vi "Analysis Configuration Dialog.vi"(11 "Data in":T1={"UI References"={"Stop Ref"=refnum, "Save Ref"=refnum, "Open Ref"=refnum, "Export Ref"=refnum, "Acquire Ref"=refnum, "Configure Ref"=refnum, "Graph Ref"=refnum, "Clear Ref"=refnum, "Analyze Ref"=refnum, "Status Ref"=refnum, "Snapshot Ref"=refnum}, "Graph Data"={"Data"=[{"t0"=timestamp(0 s since 1904-01-01), "dt"=0.001, "Y"=[0.0, 0.18799846683964833, 0.3692926533087303, 0.5374173627698757, 0.6863770400018341, 0.8108595808323735, 0.9064257689795854, 0.9696675845268409, 0.9983297385364166, 0.9913900997125904, 0.9490961449902946, 0.8729561341718822, 0.7656853233364365, 0.6311091351244097, 0.47402673897660996, 0.300039906241276, 0.11535324340830803, -0.07344707257547595, -0.25962816631122254, -0.4365505674187408, -0.5979049830575192, -0.7379372958687495, -0.8516537636065122, -0.9349991027608904, -0.9850011054694262, -0.9998766324816605, -0.9790952023238538, -0.9233979089880013, -0.8347709935146953, -0.716375011943035, -0.5724321255945906, -0.40807553307279343, -0.22916641343692226, -0.04208490860543837, 0.1464974011602751, 0.3298554148588533, 0.5014503369740866, 0.655162859793709, 0.7855113862240124, 0.887847510978669, 0.9585217890173761, 0.9950138797069145, 0.9960224255872819, 0.9615114605441677, 0.8927116924093821, 0.7920766142499667, 0.663195009476959, 0.5106629709603275, 0.33991999812206386, 0.15705501700744282, -0.03141075907812895, -0.21875638488241306, -0.39830086123182346, -0.5636413885255546, -0.7088816992555318, -0.8288423269047623, -0.9192453127499152, -0.9768667636729723, -0.9996518205634258, -0.9867879373818272, -0.9387338576538738, -0.8572032550539391, -0.7451036214770367, -0.6064325819334717, -0.44613533381770504, -0.26992829446049543, -0.0840952459318628, 0.1047367531522541, 0.28983369753066196, 0.46459477906003466, 0.6227877804881133, 0.758771324775691, 0.8676960542550545, 0.9456775653031642, 0.9899349314445249, 0.9988898749619699, 0.972223050421184, 0.9108854329621217, 0.8170644052354027, 0.6941057523695359, 0.5463943467342681, 0.37919777744325917, 0.1984785009801561, 0.010681211911579646, -0.17749698366414263, -0.3593453960058918, -0.5283790640298028, -0.6785700178191627, -0.8045622442093244, -0.9018626894832488, -0.9670014877624354, -0.9976557011314492, -0.9927321587553373, -0.9524064408346227, -0.8781166171771593, -0.7725119636778635, -0.6393584855462336, -0.483404616451529, -0.3102118829362894, -0.12595657283493283], "attributes"=variant("NI_ChannelName"=variant(string "Sine"), "NI_ExpIsRelativeTime"=variant(bool TRUE), "NI_ExpStartTimeStamp"=variant(timestamp timestamp(3405541508.232422 s since 1904-01-01)), "NI_ExpTimeStamp"=variant(timestamp timestamp(3405541508.232422 s since 1904-01-01)), "NI_ExpXDimension"=variant(string "t"))}], "Annotation List"=[], "Cursor List"=[], "Analysis Data"=[]}, "User Specified"={"Hardware Configuration"={"Physical Channel"="", "Maximum Input"=0.0, "Minimum Input"=0.0, "Sample Rate"=0.0, "Number of Samples"=0}, "Analysis Configuration"={"Statistics"=TRUE}, "New Data Behavior"=enum."Replace"}} caption="数据输入") -> (3 "Data out":T1={"UI References"={"Stop Ref"=refnum, "Save Ref"=refnum, "Open Ref"=refnum, "Export Ref"=refnum, "Acquire Ref"=refnum, "Configure Ref"=refnum, "Graph Ref"=refnum, "Clear Ref"=refnum, "Analyze Ref"=refnum, "Status Ref"=refnum, "Snapshot Ref"=refnum}, "Graph Data"={"Data"=[{"t0"=timestamp(0 s since 1904-01-01), "dt"=0.001, "Y"=[0.0, 0.18799846683964833, 0.3692926533087303, 0.5374173627698757, 0.6863770400018341, 0.8108595808323735, 0.9064257689795854, 0.9696675845268409, 0.9983297385364166, 0.9913900997125904, 0.9490961449902946, 0.8729561341718822, 0.7656853233364365, 0.6311091351244097, 0.47402673897660996, 0.300039906241276, 0.11535324340830803, -0.07344707257547595, -0.25962816631122254, -0.4365505674187408, -0.5979049830575192, -0.7379372958687495, -0.8516537636065122, -0.9349991027608904, -0.9850011054694262, -0.9998766324816605, -0.9790952023238538, -0.9233979089880013, -0.8347709935146953, -0.716375011943035, -0.5724321255945906, -0.40807553307279343, -0.22916641343692226, -0.04208490860543837, 0.1464974011602751, 0.3298554148588533, 0.5014503369740866, 0.655162859793709, 0.7855113862240124, 0.887847510978669, 0.9585217890173761, 0.9950138797069145, 0.9960224255872819, 0.9615114605441677, 0.8927116924093821, 0.7920766142499667, 0.663195009476959, 0.5106629709603275, 0.33991999812206386, 0.15705501700744282, -0.03141075907812895, -0.21875638488241306, -0.39830086123182346, -0.5636413885255546, -0.7088816992555318, -0.8288423269047623, -0.9192453127499152, -0.9768667636729723, -0.9996518205634258, -0.9867879373818272, -0.9387338576538738, -0.8572032550539391, -0.7451036214770367, -0.6064325819334717, -0.44613533381770504, -0.26992829446049543, -0.0840952459318628, 0.1047367531522541, 0.28983369753066196, 0.46459477906003466, 0.6227877804881133, 0.758771324775691, 0.8676960542550545, 0.9456775653031642, 0.9899349314445249, 0.9988898749619699, 0.972223050421184, 0.9108854329621217, 0.8170644052354027, 0.6941057523695359, 0.5463943467342681, 0.37919777744325917, 0.1984785009801561, 0.010681211911579646, -0.17749698366414263, -0.3593453960058918, -0.5283790640298028, -0.6785700178191627, -0.8045622442093244, -0.9018626894832488, -0.9670014877624354, -0.9976557011314492, -0.9927321587553373, -0.9524064408346227, -0.8781166171771593, -0.7725119636778635, -0.6393584855462336, -0.483404616451529, -0.3102118829362894, -0.12595657283493283], "attributes"=variant("NI_ChannelName"=variant(string "Sine"), "NI_ExpIsRelativeTime"=variant(bool TRUE), "NI_ExpStartTimeStamp"=variant(timestamp timestamp(3405541508.232422 s since 1904-01-01)), "NI_ExpTimeStamp"=variant(timestamp timestamp(3405541508.232422 s since 1904-01-01)), "NI_ExpXDimension"=variant(string "t"))}], "Annotation List"=[], "Cursor List"=[], "Analysis Data"=[]}, "User Specified"={"Hardware Configuration"={"Physical Channel"="", "Maximum Input"=0.0, "Minimum Input"=0.0, "Sample Rate"=0.0, "Number of Samples"=0}, "Analysis Configuration"={"Statistics"=TRUE}, "New Data Behavior"=enum."Replace"}} caption="数据输出")   [LabVIEW 2013]
doc: "当用户设置了“提示？”选项时，显示分析配置对话框。"
uses:
  controls/Data.ctl
  controls/UI References.ctl
  controls/Graph Data.ctl
  <vilib>/Utility/miscctls.llb/LVAnnotationListTypeDef.ctl
  <vilib>/Utility/miscctls.llb/LVCursorListTypeDef.ctl
  controls/User Specified Data.ctl
  controls/HW Configuration.ctl
  controls/Analysis Configuration.ctl
  controls/New Data Behavior.ctl
panel:
  # "（向上滚动可查看大型状态数据输入/输出簇）"
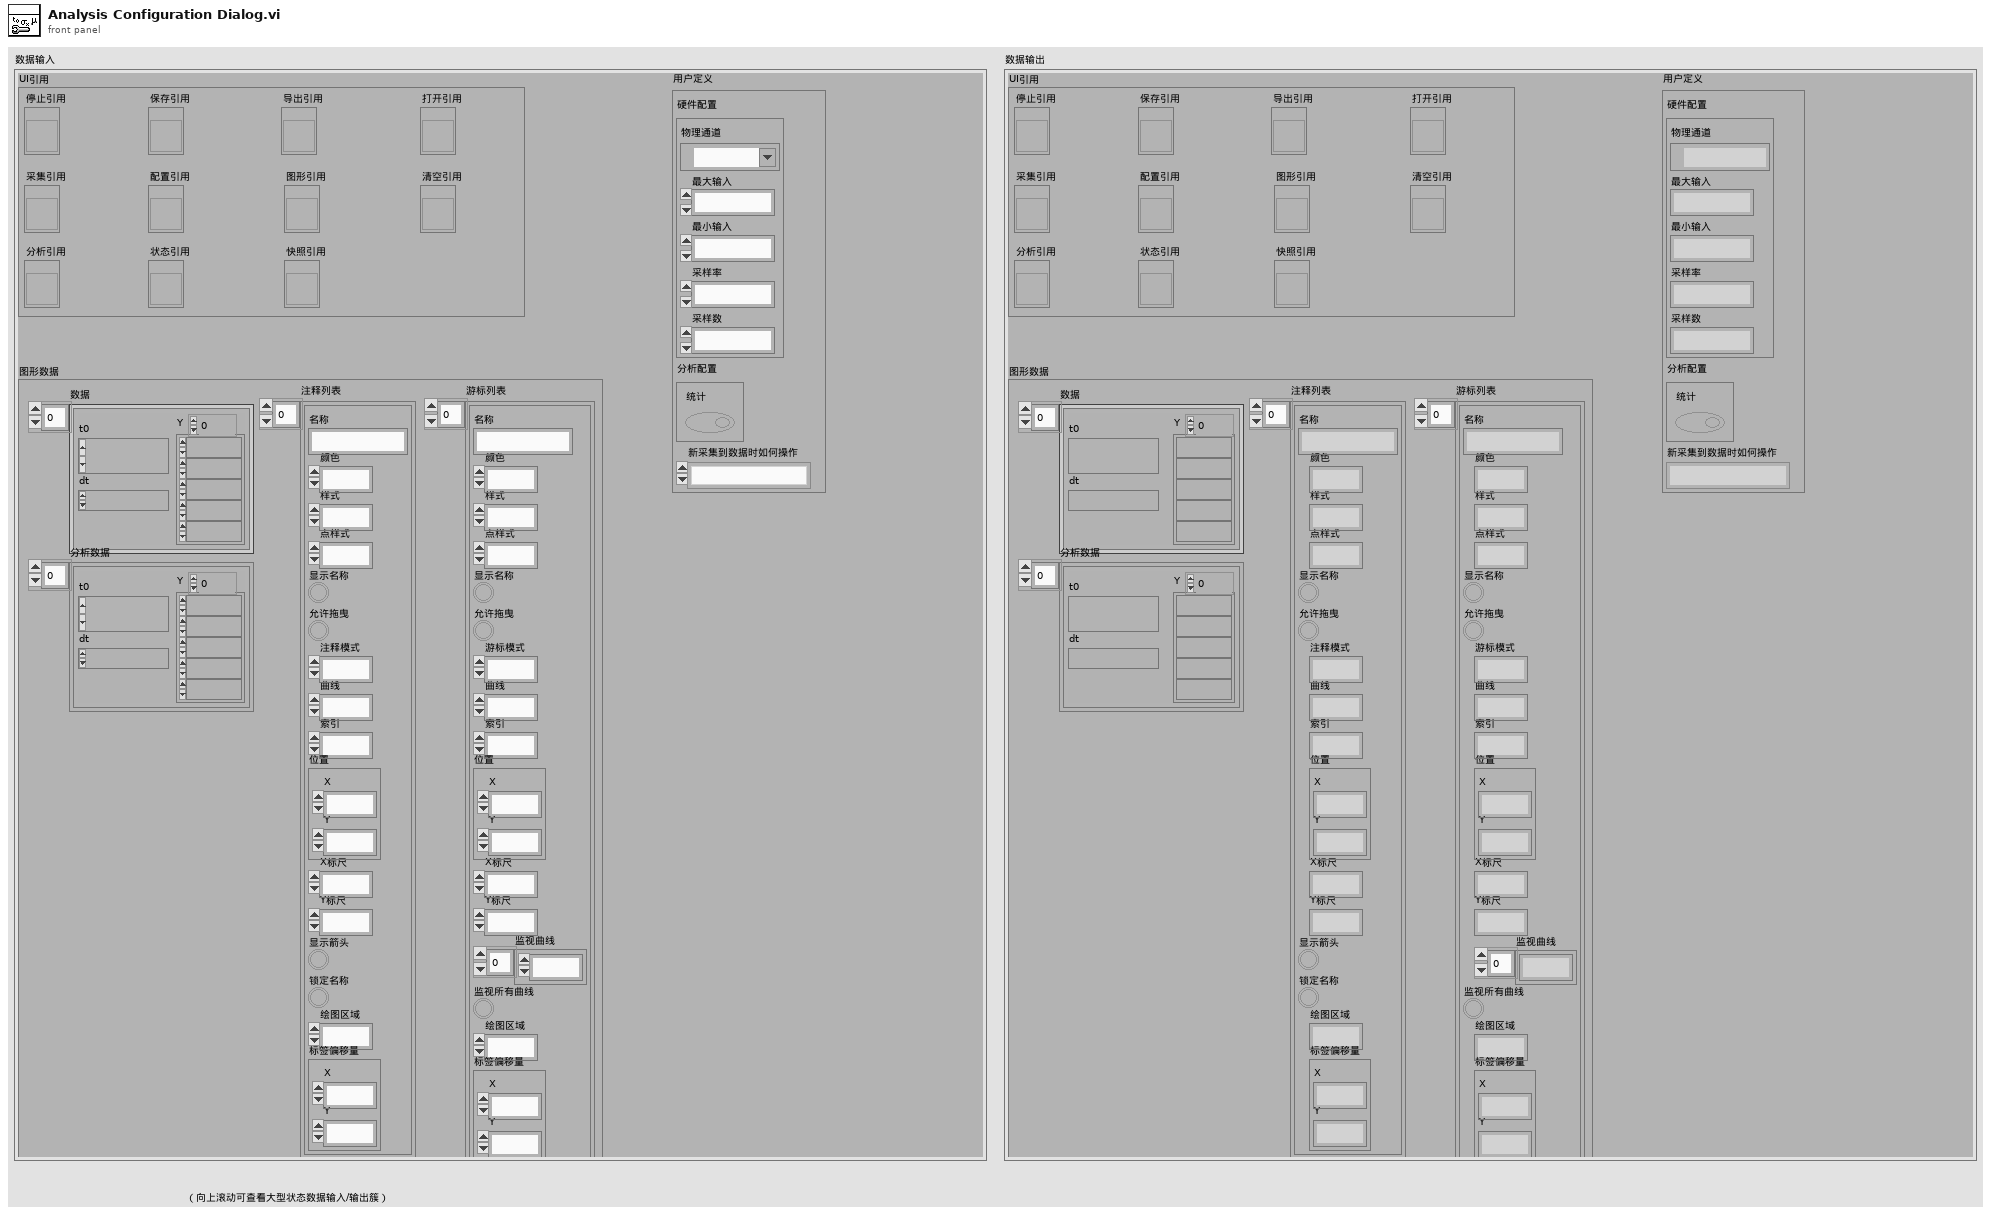
[diagram p1: front panel]
types:
  T1 = typedef "Data.ctl" = cluster{"UI References":T2, "Graph Data":T3, "User Specified":T6}
  T2 = typedef "UI References.ctl" = cluster{"Stop Ref":refnum<vi>, "Save Ref":refnum<vi>, "Open Ref":refnum<vi>, "Export Ref":refnum<vi>, "Acquire Ref":refnum<vi>, "Configure Ref":refnum<vi>, "Graph Ref":refnum<vi>, "Clear Ref":refnum<vi>, "Analyze Ref":refnum<vi>, "Status Ref":refnum<vi>, "Snapshot Ref":refnum<vi>}
  T3 = typedef "Graph Data.ctl" = cluster{"Data":waveform(dbl)[], "Annotation List":T4, "Cursor List":T5, "Analysis Data":waveform(dbl)[]}
  T4 = typedef "LVAnnotationListTypeDef.ctl" = cluster{"Name":string, "Color":u32, "Style":u8, "Point Style":u8, "Name Visible":bool, "Allow Drag":bool, "Annotation Mode":u32, "Plot":i32, "Index":i32, "Position":cluster{"X":dbl, "Y":dbl}, "X Scale":u32, "Y Scale":u32, "Show Arrow":bool, "Lock Name":bool, "Plot Area":i32, "Label Offset":cluster{"X":dbl, "Y":dbl}}[]
  T5 = typedef "LVCursorListTypeDef.ctl" = cluster{"Name":string, "Color":u32, "Style":u8, "Point Style":u8, "Name Visible":bool, "Allow Drag":bool, "Cursor Mode":u32, "Plot":i32, "Index":i32, "Position":cluster{"X":dbl, "Y":dbl}, "X Scale":u32, "Y Scale":u32, "Watch Plots":i32[], "Watch All Plots":bool, "Plot Area":i32, "Label Offset":cluster{"X":dbl, "Y":dbl}}[]
  T6 = typedef "User Specified Data.ctl" = cluster{"Hardware Configuration":T7, "Analysis Configuration":T8, "New Data Behavior":T9}
  T7 = typedef "HW Configuration.ctl" = cluster{"Physical Channel":tag, "Maximum Input":dbl, "Minimum Input":dbl, "Sample Rate":dbl, "Number of Samples":i32}
  T8 = typedef "Analysis Configuration.ctl" = cluster{"Statistics":bool}
  T9 = typedef "New Data Behavior.ctl" = enum16{"Replace", "Overlay", "Append"}
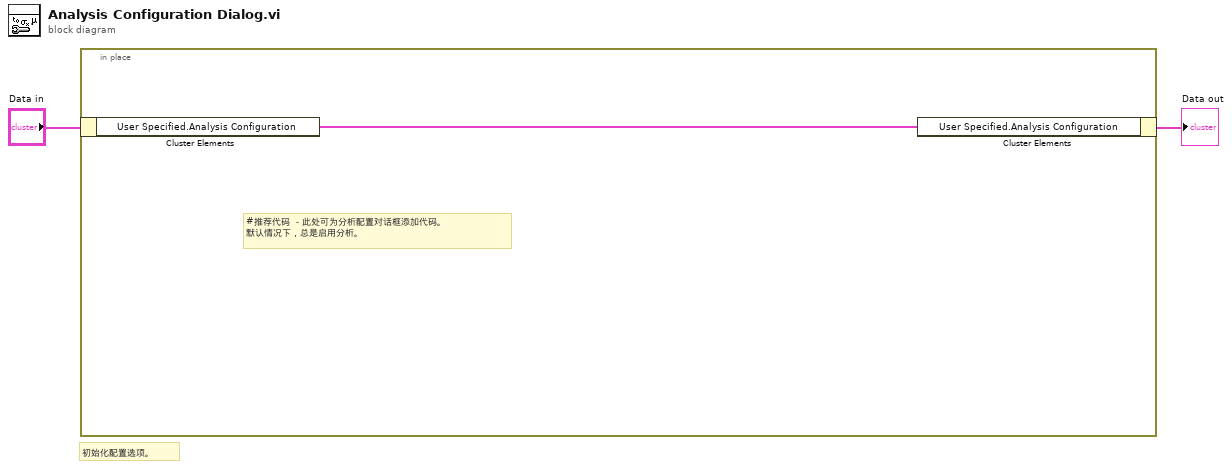
[diagram p0: block diagram]
diagram:
  # "初始化配置选项。"
  n1 = in-place {
    # "#推荐代码 －此处可为分析配置对话框添加代码。\n默认情况下，总是启用分析。"
    n2 = in-place-cluster #1("Data in") -> ("User Specified.Analysis Configuration"=w3:T8)
    n3 = in-place-cluster #1("User Specified.Analysis Configuration"=w3) -> (→"Data out":T1)
  }
